vi "ep_3-Phase SVAF.vi"(0 "phase A":dbl[](array[numeric]), 1 "reset? (F)":bool, 2 "difference? (T)":bool=TRUE, 5 "phase B":dbl[](array[numeric]), 7 "phase C":dbl[](array[numeric]), 11 "error in (no error)":errorcluster, 12 "previous SVAF state":T1) -> (4 "SVAF signal":dbl[](array[numeric]), 14 "next SVAF state":T1, 15 "error out":errorcluster)   [LabVIEW 2014, in "NI_EP_Motor Monitoring.lvlib"]
uses:
  <vilib>/addons/Electrical Power/Motor Monitoring/NI_EP_Motor Monitoring.lvlib
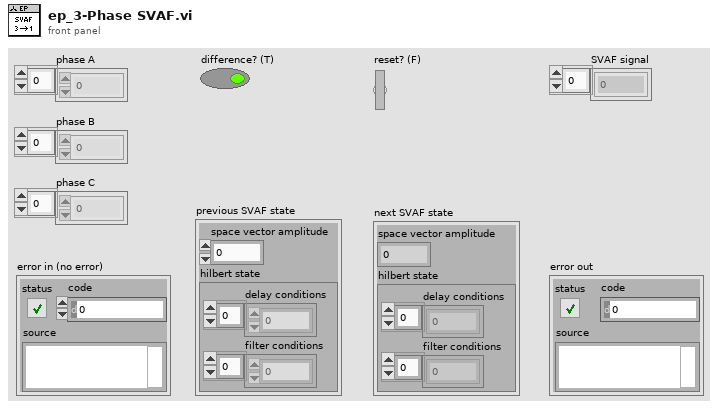
[diagram p1: front panel]
types:
  T1 = cluster{"space vector amplitude":dbl, "hilbert state":cluster{"delay conditions":dbl[], "filter conditions":dbl[]}}
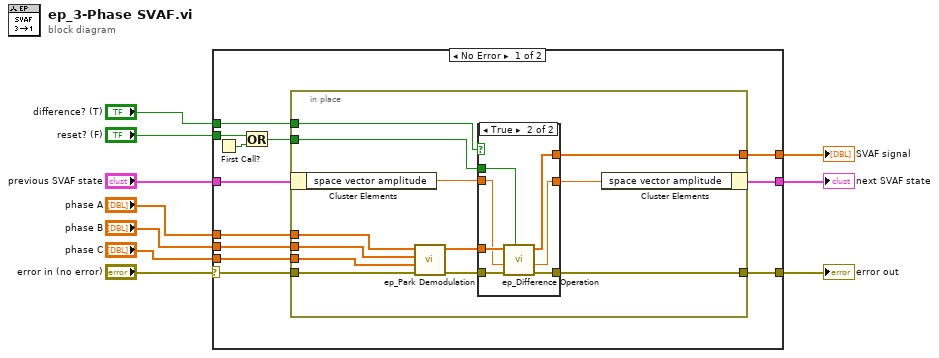
[diagram p0: block diagram]
diagram:
  n1 = case shown="No Error" "error in (no error)" {
    selector: "error in (no error)" -> [w18 w44]
    tunnel: [w13 w44] -> w9
    tunnel: "phase A" -> [w22 _]
    tunnel: "phase B" -> [w21 _]
    tunnel: "phase C" -> [w20 _]
    tunnel: [w19 _] -> w5
    tunnel: "reset? (F)" -> [w16 _]
    tunnel: "difference? (T)" -> [w14 _]
    tunnel: "previous SVAF state" -> [w12 _]
    tunnel: [w11 _] -> w1
    frame No Error {
      n2 = First Call?() -> (First Call?: T/F=w17:bool)
      n3 = Or(x=w16, y=w17) -> (x .or. y?=w15:bool)
      n4 = in-place {
        in-place-border: w22 -> [w34]
        in-place-border: w21 -> [w33]
        in-place-border: w20 -> [w32]
        in-place-border: [w30] -> w19
        in-place-border: w18 -> [w29]
        in-place-border: w15 -> [w28]
        in-place-border: w14 -> [w27]
        in-place-border: [w25] -> w13
        n5 = in-place-cluster #1(w12) -> ("space vector amplitude"=w24:dbl)
        n6 = call <vilib>:"ep_Park Demodulation.vi"("error in (no error)"=w29, "phase C"=w32, "phase B"=w33, "phase A"=w34) -> ("error out"=w26:errorcluster, "demodulated signal"=w31:dbl[])  [unwired: 6 in]
        n7 = case shown="True" w27 {
          tunnel: [_ w39] -> w23
          tunnel: w24 -> [_ w41]
          tunnel: w31 -> [w36 w42]
          tunnel: [w36 w40] -> w30
          tunnel: w28 -> [_ w43]
          tunnel: w26 -> [w35 w38]
          tunnel: [w35 w37] -> w25
          frame False {
          }
          frame True {
            n8 = call <vilib>:"ep_Difference Operation.vi"("reset? (F)"=w43, "error in (no error)"=w38, "previous value"=w41, "signal in"=w42) -> ("error out"=w37:errorcluster, "next  value"=w39:dbl, "signal out"=w40:dbl[])  [unwired: 5 in]
          }
        }
        n9 = in-place-cluster #1("space vector amplitude"=w23) -> (w11:T1)
      }
    }
    frame Error {
    }
  }
  "error out" <- w9
  "SVAF signal" <- w5
  "next SVAF state" <- w1
